vi "Get Reentrant.vi"(8 "error in (no error)":errorcluster, 11 "measurement in":refnum<class "Continuous Counting Measurement.lvclass">) -> (0 "error out":errorcluster, 2 "reentrant":bool, 3 "measurement out":refnum<class "Continuous Counting Measurement.lvclass">)   [LabVIEW 2021, in "MeasurementServerTests.lvlib" / "Measurement Service Tests.lvlib" / "Continuous Counting Measurement.lvclass"]
uses:
  Continuous Counting Measurement.lvclass
  Continuous Counting Measurement.lvclass/Continuous Counting Measurement.ctl
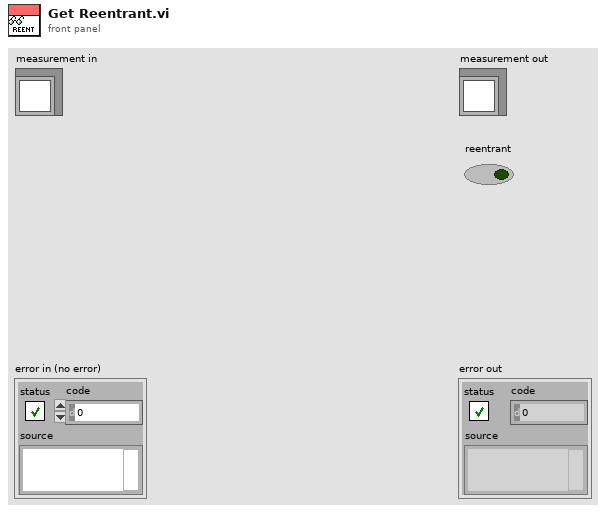
[diagram p1: front panel]
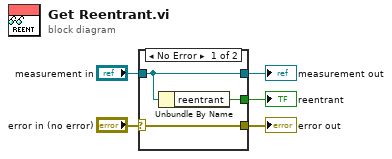
[diagram p0: block diagram]
diagram:
  n1 = case shown="No Error" "error in (no error)" {
    selector: "error in (no error)" -> [w8 w9]
    tunnel: [w8 w9] -> w4
    tunnel: [w7 w10] -> w2
    tunnel: "measurement in" -> [w7 w10]
    tunnel: [w6 _] -> w1
    frame No Error {
      n2 = Unbundle By Name(w7) -> ("reentrant"=w6:bool)
    }
    frame Error {
    }
  }
  "error out" <- w4
  "measurement out" <- w2
  "reentrant" <- w1
